vi "BODE_AUTO_v9.vi"() -> ()   [LabVIEW 2015]
uses:
  <vilib>/Analysis/1siggen.llb/Ramp Pattern by Samples.vi
  <vilib>/Utility/file.llb/Write Delimited Spreadsheet (DBL).vi
  <vilib>/Utility/file.llb/Write Delimited Spreadsheet (string).vi
  <vilib>/Analysis/NI_AALBase.lvlib
panel:
  out "Measurement Type":string="S21"
  out "Sweeps Waiting To Be Saved":i32(knob) scale=0.0..15.0
  out "Approximate Sweep Time (s)":sgl
  out "Iterations":i32
  in  "Path to Folder (create new folder for test)":path
  out "Start Time and Date":timestamp
  in  "File Name for Collected Sound Data":string="TestName"
  out "S21 Transmission Sweep":cluster{"Ramp Pattern":dbl[], dbl[]}(graph)
  in  "Stop Testing":bool
  out "Collecting Data":bool
  out "Set":bool
  out "Testing Parameters Set":string
  in  "Source Power (max 13dBm)":string="0"
  in  "Reciever Bandwidth (Hz)":string="300"
  in  "Number of Points":string="50"
  in  "End Frequency (Hz) (max 40MHz)":string="6000000"
  in  "Start Frequency (Hz) (100Hz)":string="1000000"
  out "Device Identification":string
  in  "TCPIP0::<IP_AD>::<PORT>:SOCKET":refnum<visa-resource-name>
  # "CLICK ONLY ONCE\nIt takes time as all loops need to complete and all data must be saved."
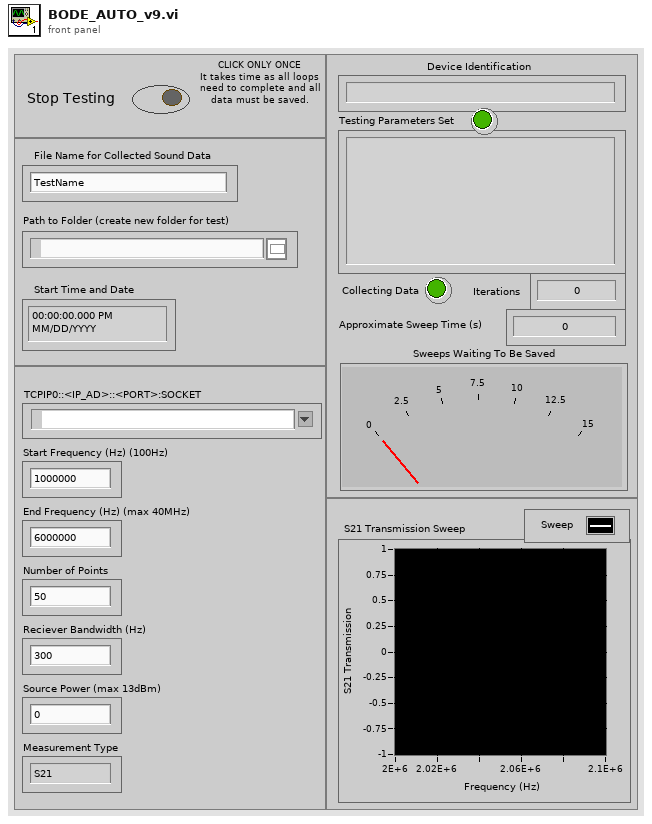
[diagram p1: front panel]
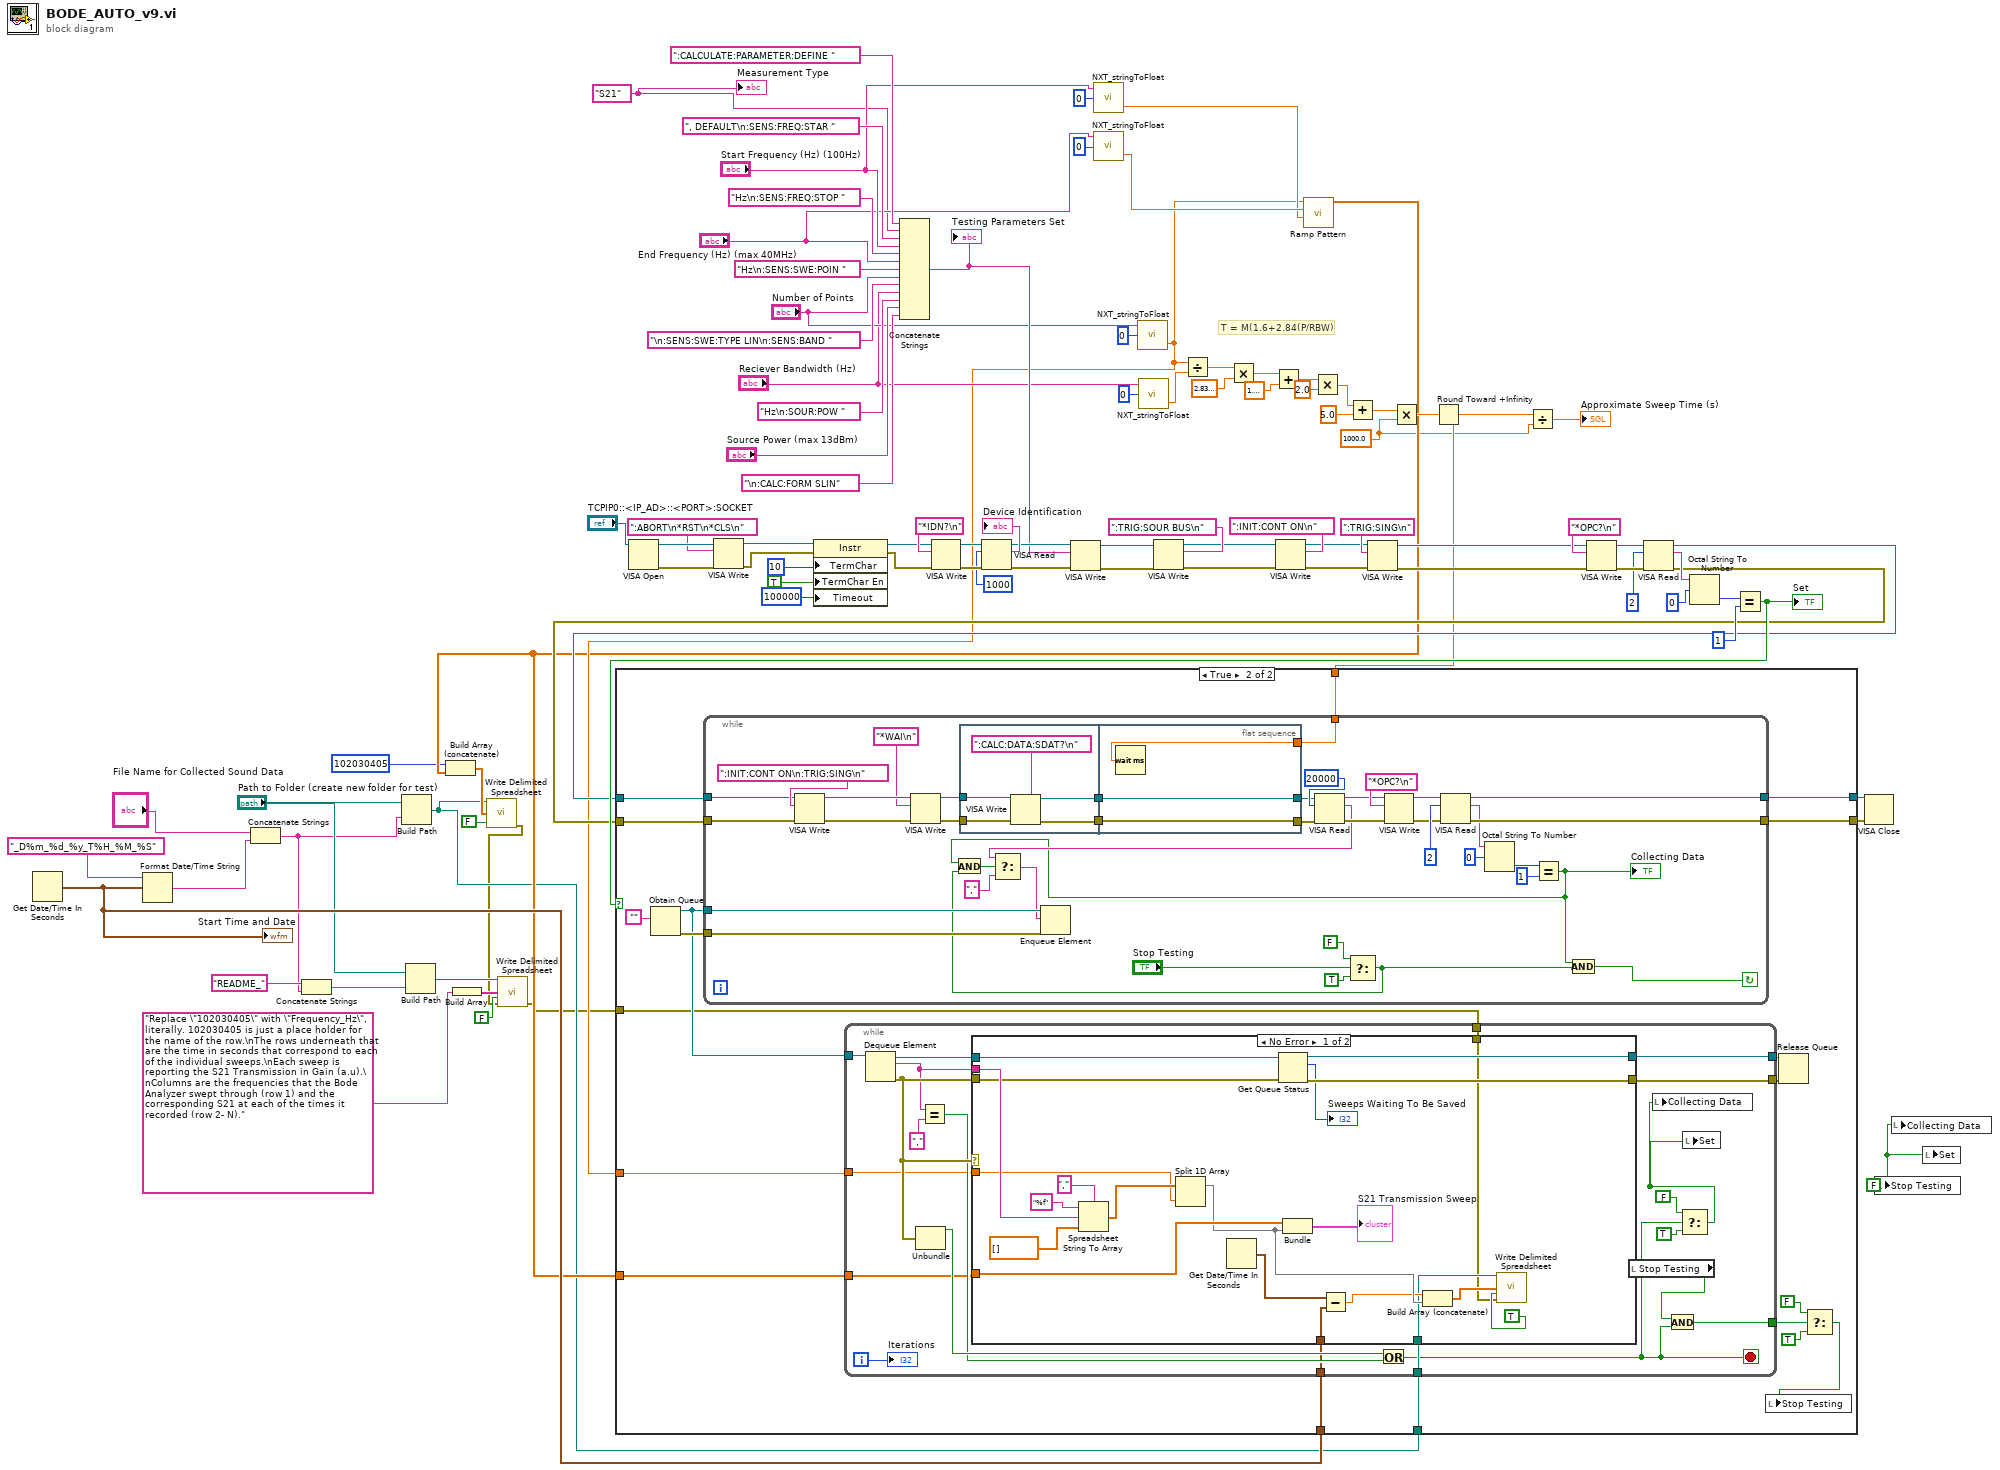
[diagram p0: block diagram]
diagram:
  w3 = "S21" ("Measurement Type 2")
  w4 = FALSE ("STOP")
  w5 = sgl 1000.0 ("y")
  # "T = M(1.6+2.84(P/RBW)"
  n1 = Get Date/Time In Seconds() -> (seconds since 1Jan1904=w20:timestamp)
  "Start Time and Date" <- w20
  n2 = Format Date/Time String(time format string (%c)="_D%m_%d_%y_T%H_%M_%S", seconds (now)=w20) -> (date/time string=w21:string)  [unwired: 1 in]
  n3 = Concatenate Strings("File Name for Collected Sound Data", w21) -> (w13:string)
  n4 = Concatenate Strings("README_" ("string"), w13) -> (w15:string)
  n5 = Build Path(base path="Path to Folder (create new folder for test)", name or relative path=w13) -> (appended path=w17:path)
  n6 = Build Path(base path="Path to Folder (create new folder for test)", name or relative path=w15) -> (appended path=w12:path)
  n7 = Build Array("Replace \"102030405\" with \"Frequency_Hz\", literally. 102030405 is just a place holder for the name of the row.\nThe rows underneath that are the time in seconds that correspond to each of the individual sweeps.\nEach sweep is reporting the S21 Transmission in Gain (a.u).\nColumns are the frequencies that the Bode Analyzer swept through (row 1) and the corresponding S21 at each of the times it recorded (row 2- N)." ("string")) -> (w10:string[])
  n8 = VISA Open(VISA resource name="TCPIP0::<IP_AD>::<PORT>:SOCKET") -> (VISA resource name=w68:refnum<visa-resource-name>, error out=w69:errorcluster)  [unwired: 4 in]
  n9 = VISA Write(VISA resource name=w68, write buffer=":ABORT\n*RST\n*CLS\n", error in (no error)=w69) -> (VISA resource name out=w67:refnum<visa-resource-name>, error out=w66:errorcluster)  [unwired: 1 out]
  n10 = property class="Instr"(reference=w67, error in=w66, "TermChar"=u8 10 ("Message Based Settings:Termination Character"), "TermChar En"=TRUE ("Message Based Settings:Termination Character Enable"), "Timeout"=u32 100000 ("General Settings:Timeout Value")) -> (reference out=w73:refnum<visa-resource-name>, error out=w72:errorcluster)
  n11 = Concatenate Strings(":CALCULATE:PARAMETER:DEFINE " ("string"), w3, ", DEFAULT\n:SENS:FREQ:STAR " ("string"), "Start Frequency (Hz) (100Hz)", "Hz\n:SENS:FREQ:STOP " ("string"), "End Frequency (Hz) (max 40MHz)", "Hz\n:SENS:SWE:POIN " ("string"), "Number of Points", "\n:SENS:SWE:TYPE LIN\n:SENS:BAND " ("string"), "Reciever Bandwidth (Hz)", "Hz\n:SOUR:POW " ("string"), "Source Power (max 13dBm)", "\n:CALC:FORM SLIN" ("string")) -> (w57:string)
  "Testing Parameters Set" <- w57
  n12 = VISA Write(VISA resource name=w73, write buffer="*IDN?\n", error in (no error)=w72) -> (VISA resource name out=w94:refnum<visa-resource-name>, error out=w95:errorcluster)  [unwired: 1 out]
  n13 = VISA Read(VISA resource name=w94, byte count=u32 1000, error in (no error)=w95) -> (VISA resource name out=w60:refnum<visa-resource-name>, read buffer=→"Device Identification":string, error out=w61:errorcluster)  [unwired: 1 out]
  n14 = VISA Write(VISA resource name=w60, write buffer=w57, error in (no error)=w61) -> (VISA resource name out=w59:refnum<visa-resource-name>, error out=w58:errorcluster)  [unwired: 1 out]
  n15 = call <vilib>:"NXT_stringToFloat.vi"("offset"=0, "string"="Start Frequency (Hz) (100Hz)") -> ("number"=w27:sgl)  [unwired: 1 in, 1 out]
  n16 = call <vilib>:"NXT_stringToFloat.vi"("offset"=0, "string"="End Frequency (Hz) (max 40MHz)") -> ("number"=w28:sgl)  [unwired: 1 in, 1 out]
  n17 = call <vilib>:"NXT_stringToFloat.vi"("offset"=0, "string"="Number of Points") -> ("number"=w25:sgl)  [unwired: 1 in, 1 out]
  n18 = call <vilib>:"NXT_stringToFloat.vi"("offset"=0, "string"="Reciever Bandwidth (Hz)") -> ("number"=w42:sgl)  [unwired: 1 in, 1 out]
  n19 = VISA Write(VISA resource name=w59, write buffer=":TRIG:SOUR BUS\n", error in (no error)=w58) -> (VISA resource name out=w81:refnum<visa-resource-name>, error out=w80:errorcluster)  [unwired: 1 out]
  n20 = Divide(x=w25, y=w42) -> (x/y=w41:sgl)
  n21 = Multiply(x=w41, y=sgl 2.84) -> (x*y=w39:sgl)
  n22 = Add(x=w39, y=sgl 1.6) -> (x+y=w37:sgl)
  n23 = VISA Write(VISA resource name=w81, write buffer=":INIT:CONT ON\n", error in (no error)=w80) -> (VISA resource name out=w79:refnum<visa-resource-name>, error out=w78:errorcluster)  [unwired: 1 out]
  n24 = call-poly <vilib>:"Ramp Pattern.vi"("start"=w27, "end"=w28, "samples"=w25) -> ("Ramp Pattern"=w19:dbl[])  [unwired: 7 in, 1 out]
  n25 = Build Array (concatenate)(102030405 ("offset"), w19) -> (w18:dbl[])
  n26 = call-poly <vilib>:"Write Delimited Spreadsheet.vi"("file path (dialog if empty)"=w17, "1D data"=w18, "append to file? (F)"=FALSE ("append to file? (new file:F)")) -> ("error out"=w2:errorcluster)  [unwired: 11 in, 1 out]
  n27 = call-poly <vilib>:"Write Delimited Spreadsheet.vi"("file path (dialog if empty)"=w12, "1D data"=w10, "append to file? (F)"=FALSE ("append to file? (new file:F)"), "error in (no error)"=w2) -> ("error out"=w1:errorcluster)  [unwired: 10 in, 1 out]
  n28 = Multiply(x=w37, y=sgl 2.0) -> (x*y=w35:sgl)
  n29 = Add(x=w35, y=sgl 5.0) -> (x+y=w33:sgl)
  n30 = VISA Write(VISA resource name=w79, write buffer=":TRIG:SING\n", error in (no error)=w78) -> (VISA resource name out=w71:refnum<visa-resource-name>, error out=w70:errorcluster)  [unwired: 1 out]
  n31 = Multiply(x=w33, y=w5) -> (x*y=w26:sgl)
  n32 = Round Toward +Infinity(x=w26) -> (ceil(x): smallest int >= x=w6:sgl)
  n33 = Divide(x=w6, y=w5) -> (x/y=→"Approximate Sweep Time (s)":sgl)
  n34 = VISA Write(VISA resource name=w71, write buffer="*OPC?\n", error in (no error)=w70) -> (VISA resource name out=w63:refnum<visa-resource-name>, error out=w64:errorcluster)  [unwired: 1 out]
  n35 = VISA Read(VISA resource name=w63, byte count=u32 2, error in (no error)=w64) -> (VISA resource name out=w50:refnum<visa-resource-name>, read buffer=w56:string, error out=w49:errorcluster)  [unwired: 1 out]
  n36 = Octal String To Number(3:0 ("offset"), 4:w56) -> (0:w54:u32)  [unwired: 1 in, 1 out]
  n37 = Equal?(x=w54, y=u32 1) -> (x = y?=w52:bool)
  "Set" <- w52
  n38 = case shown="True" w52 {
    tunnel: w50 -> [w99 w117]
    tunnel: w49 -> [w98 w118]
    tunnel: [w99 w116] -> w48
    tunnel: [w98 w115] -> w47
    tunnel: w6 -> [_ w109]
    tunnel: w19 -> [_ w108]
    tunnel: w25 -> [_ w107]
    tunnel: w20 -> [_ w106]
    tunnel: w17 -> [_ w105]
    tunnel: w1 -> [_ w100]
    frame False {
    }
    frame True {
      n39 = Obtain Queue(element data type="") -> (queue out=w112:refnum<queue>, error out=w114:errorcluster)  [unwired: 4 in, 1 out]
      n40 = while {
        tunnel: w118 -> [w182]
        tunnel: w117 -> [w181]
        tunnel: [w180] -> w116
        tunnel: [w179] -> w115
        tunnel: w112 -> [w178]
        tunnel: w114 -> [w177]
        tunnel: w109 -> [w165]
        stop <- w164 continue-if-true
        n41 = VISA Write(VISA resource name=w181, write buffer=":INIT:CONT ON\n:TRIG:SING\n", error in (no error)=w182) -> (VISA resource name out=w197:refnum<visa-resource-name>, error out=w198:errorcluster)  [unwired: 1 out]
        n42 = VISA Write(VISA resource name=w197, write buffer="*WAI\n", error in (no error)=w198) -> (VISA resource name out=w195:refnum<visa-resource-name>, error out=w196:errorcluster)  [unwired: 1 out]
        n43 = flat-sequence {
          tunnel: w196 -> [w204]
          tunnel: w195 -> [w203]
          tunnel: [w202] -> w167
          tunnel: [w201] -> w166
          tunnel: [w207] -> w193
          tunnel: [w208] -> w194
          tunnel: w167 -> [w208]
          tunnel: w166 -> [w207]
          tunnel: w165 -> [w206]
          frame #0 {
            n44 = VISA Write(VISA resource name=w203, write buffer=":CALC:DATA:SDAT?\n", error in (no error)=w204) -> (VISA resource name out=w201:refnum<visa-resource-name>, error out=w202:errorcluster)  [unwired: 1 out]
          }
          frame #1 {
            n45 = Wait (ms)(milliseconds to wait=w206) -> ()  [unwired: 1 out]
          }
        }
        n46 = VISA Read(VISA resource name=w193, byte count=u32 20000, error in (no error)=w194) -> (VISA resource name out=w184:refnum<visa-resource-name>, read buffer=w169:string, error out=w183:errorcluster)  [unwired: 1 out]
        n47 = Select(t=FALSE, s="Stop Testing", f=TRUE) -> (s? t:f=w171:bool)
        n48 = VISA Write(VISA resource name=w184, write buffer="*OPC?\n", error in (no error)=w183) -> (VISA resource name out=w187:refnum<visa-resource-name>, error out=w186:errorcluster)  [unwired: 1 out]
        n49 = VISA Read(VISA resource name=w187, byte count=u32 2, error in (no error)=w186) -> (VISA resource name out=w180:refnum<visa-resource-name>, read buffer=w176:string, error out=w179:errorcluster)  [unwired: 1 out]
        n50 = Octal String To Number(3:0 ("offset"), 4:w176) -> (0:w189:u32)  [unwired: 1 in, 1 out]
        n51 = Equal?(x=w189, y=u32 1) -> (x = y?=w163:bool)
        "Collecting Data" <- w163
        n52 = And(x=w163, y=w171) -> (x .and. y?=w172:bool)
        n53 = Select(t=w169, s=w172, f="," ("delimiter (Tab)")) -> (s? t:f=w168:string)
        n54 = Enqueue Element(queue=w178, element=w168, error in (no error)=w177) -> ()  [unwired: 1 in, 3 out]
        n55 = And(x=w163, y=w171) -> (x .and. y?=w164:bool)
      }
      n56 = while {
        tunnel: [w138] -> w111
        tunnel: [w137] -> w110
        tunnel: w112 -> [w136]
        tunnel: w108 -> [w130]
        tunnel: w107 -> [w129]
        tunnel: w106 -> [w128]
        tunnel: w105 -> [w127]
        tunnel: [w120] -> w102
        tunnel: w100 -> [w119]
        i -> [w126]
        stop <- w121 stop-if-true
        n57 = Dequeue Element(queue=w136) -> (queue out=w139:refnum<queue>, element=w133:string, error out=w135:errorcluster)  [unwired: 2 in, 1 out]
        n58 = Unbundle(w135) -> ("status"=w134:bool)  [unwired: 2 out]
        n59 = Equal?(x=w133, y="," ("delimiter (Tab)")) -> (x = y?=w131:bool)
        n60 = case shown="No Error" w135 {
          tunnel: w133 -> [w157 _]
          tunnel: w139 -> [w156 w162]
          tunnel: w135 -> [w155 w161]
          tunnel: [w154 w162] -> w138
          tunnel: [w153 w161] -> w137
          tunnel: w130 -> [w152 _]
          tunnel: w129 -> [w149 _]
          tunnel: w128 -> [w147 _]
          tunnel: w127 -> [w142 _]
          tunnel: w119 -> [w140 _]
          frame No Error {
            n61 = Spreadsheet String To Array(delimiter (Tab)=",", format string="%f", spreadsheet string=w157, array type (2D Dbl)=dbl[] []) -> (array=w150:dbl[])
            n62 = Split 1D Array(array=w150, index=w149) -> (first subarray=w146:dbl[])  [unwired: 1 out]
            n63 = Get Date/Time In Seconds() -> (seconds since 1Jan1904=w148:timestamp)
            n64 = Get Queue Status(queue=w156, error in (no error)=w155) -> (queue out=w154:refnum<queue>, # pending remove=→"Sweeps Waiting To Be Saved":i32, error out=w153:errorcluster)  [unwired: 1 in, 5 out]
            n65 = Bundle("Ramp Pattern"=w152, w146) -> (→"S21 Transmission Sweep":cluster{"Ramp Pattern":dbl[], dbl[]})  [unwired: 1 in]
            n66 = Subtract(x=w148, y=w147) -> (x-y=w144:dbl)
            n67 = Build Array (concatenate)(w144, w146) -> (w143:dbl[])
            n68 = call-poly <vilib>:"Write Delimited Spreadsheet.vi"("file path (dialog if empty)"=w142, "1D data"=w143, "append to file? (F)"=TRUE ("append to file? (new file:F)"), "error in (no error)"=w140) -> ()  [unwired: 10 in, 2 out]
          }
          frame Error {
          }
        }
        n69 = Or(x=w134, y=w131) -> (x .or. y?=w121:bool)
        n70 = local read "Stop Testing"() -> (w122:bool)
        n71 = And(x=w122, y=w121) -> (x .and. y?=w120:bool)
        n72 = Select(t=FALSE, s=w121, f=TRUE) -> (s? t:f=w123:bool)
        n73 = local write "Collecting Data"(w123) -> ()
        n74 = local write "Set"(w123) -> ()
        "Iterations" <- w126
      }
      n75 = Release Queue(queue=w111, error in (no error)=w110) -> ()  [unwired: 1 in, 3 out]
      n76 = Select(t=FALSE, s=w102, f=TRUE) -> (s? t:f=w101:bool)
      n77 = local write "Stop Testing"(w101) -> ()
    }
  }
  n78 = VISA Close(VISA resource name=w48, error in (no error)=w47) -> ()  [unwired: 1 out]
  n79 = local write "Stop Testing"(w4) -> ()
  n80 = local write "Collecting Data"(w4) -> ()
  n81 = local write "Set"(w4) -> ()
  "Measurement Type" <- w3
